vi "Message Types.vi"(8 "error in (no error)":errorcluster, 11 "MessageTransformer in":refnum<class "MessageTransformer.lvclass">) -> (0 "error out":errorcluster, 2 "Message Types":string[](array[string]), 3 "MessageTransformer out":refnum<class "MessageTransformer.lvclass">)   [LabVIEW 2020, in "Volatus.lvlib" / "MessageTransformer.lvclass"]
uses:
  MessageTransformer.lvclass
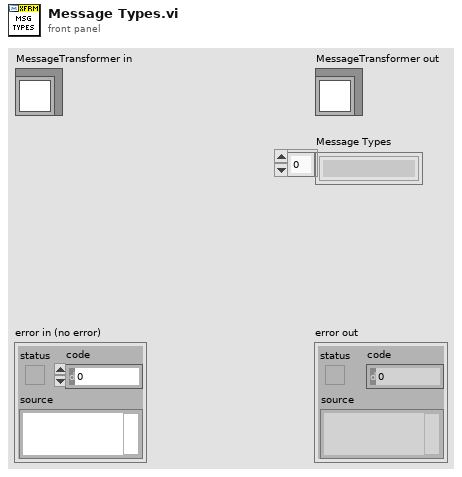
[diagram p1: front panel]
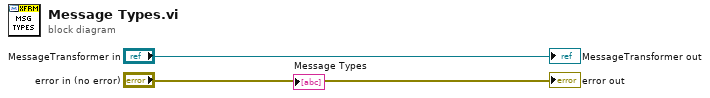
[diagram p0: block diagram]
diagram:
  "error out" <- "error in (no error)"
  "MessageTransformer out" <- "MessageTransformer in"
